vi "TDMS_Open - 1D.vi"(7 "Offset":bool, 8 "Gate 2":dbl=15.0, 9 "Gate 1":dbl=5.0, 10 "Input 2D":dbl[][](array[numeric]), 11 "Open":bool) -> (1 "Output 2D":dbl[][](array[numeric]), 3 "Freq_Sampling_SizeX_SizeY":dbl[](array[numeric]))   [LabVIEW 2018]
uses:
  <vilib>/Platform/NI_3dgraph.lvlib
panel:
  in  "milliseconds to wait":u32
  in  "3D Surface":refnum<k7>(container)
  in  "Samples per Channel":i32=1000 caption="Samples"
  in  "Rate":dbl=60000.0 caption="Sample Rate (Hz)" format="%0.0f"
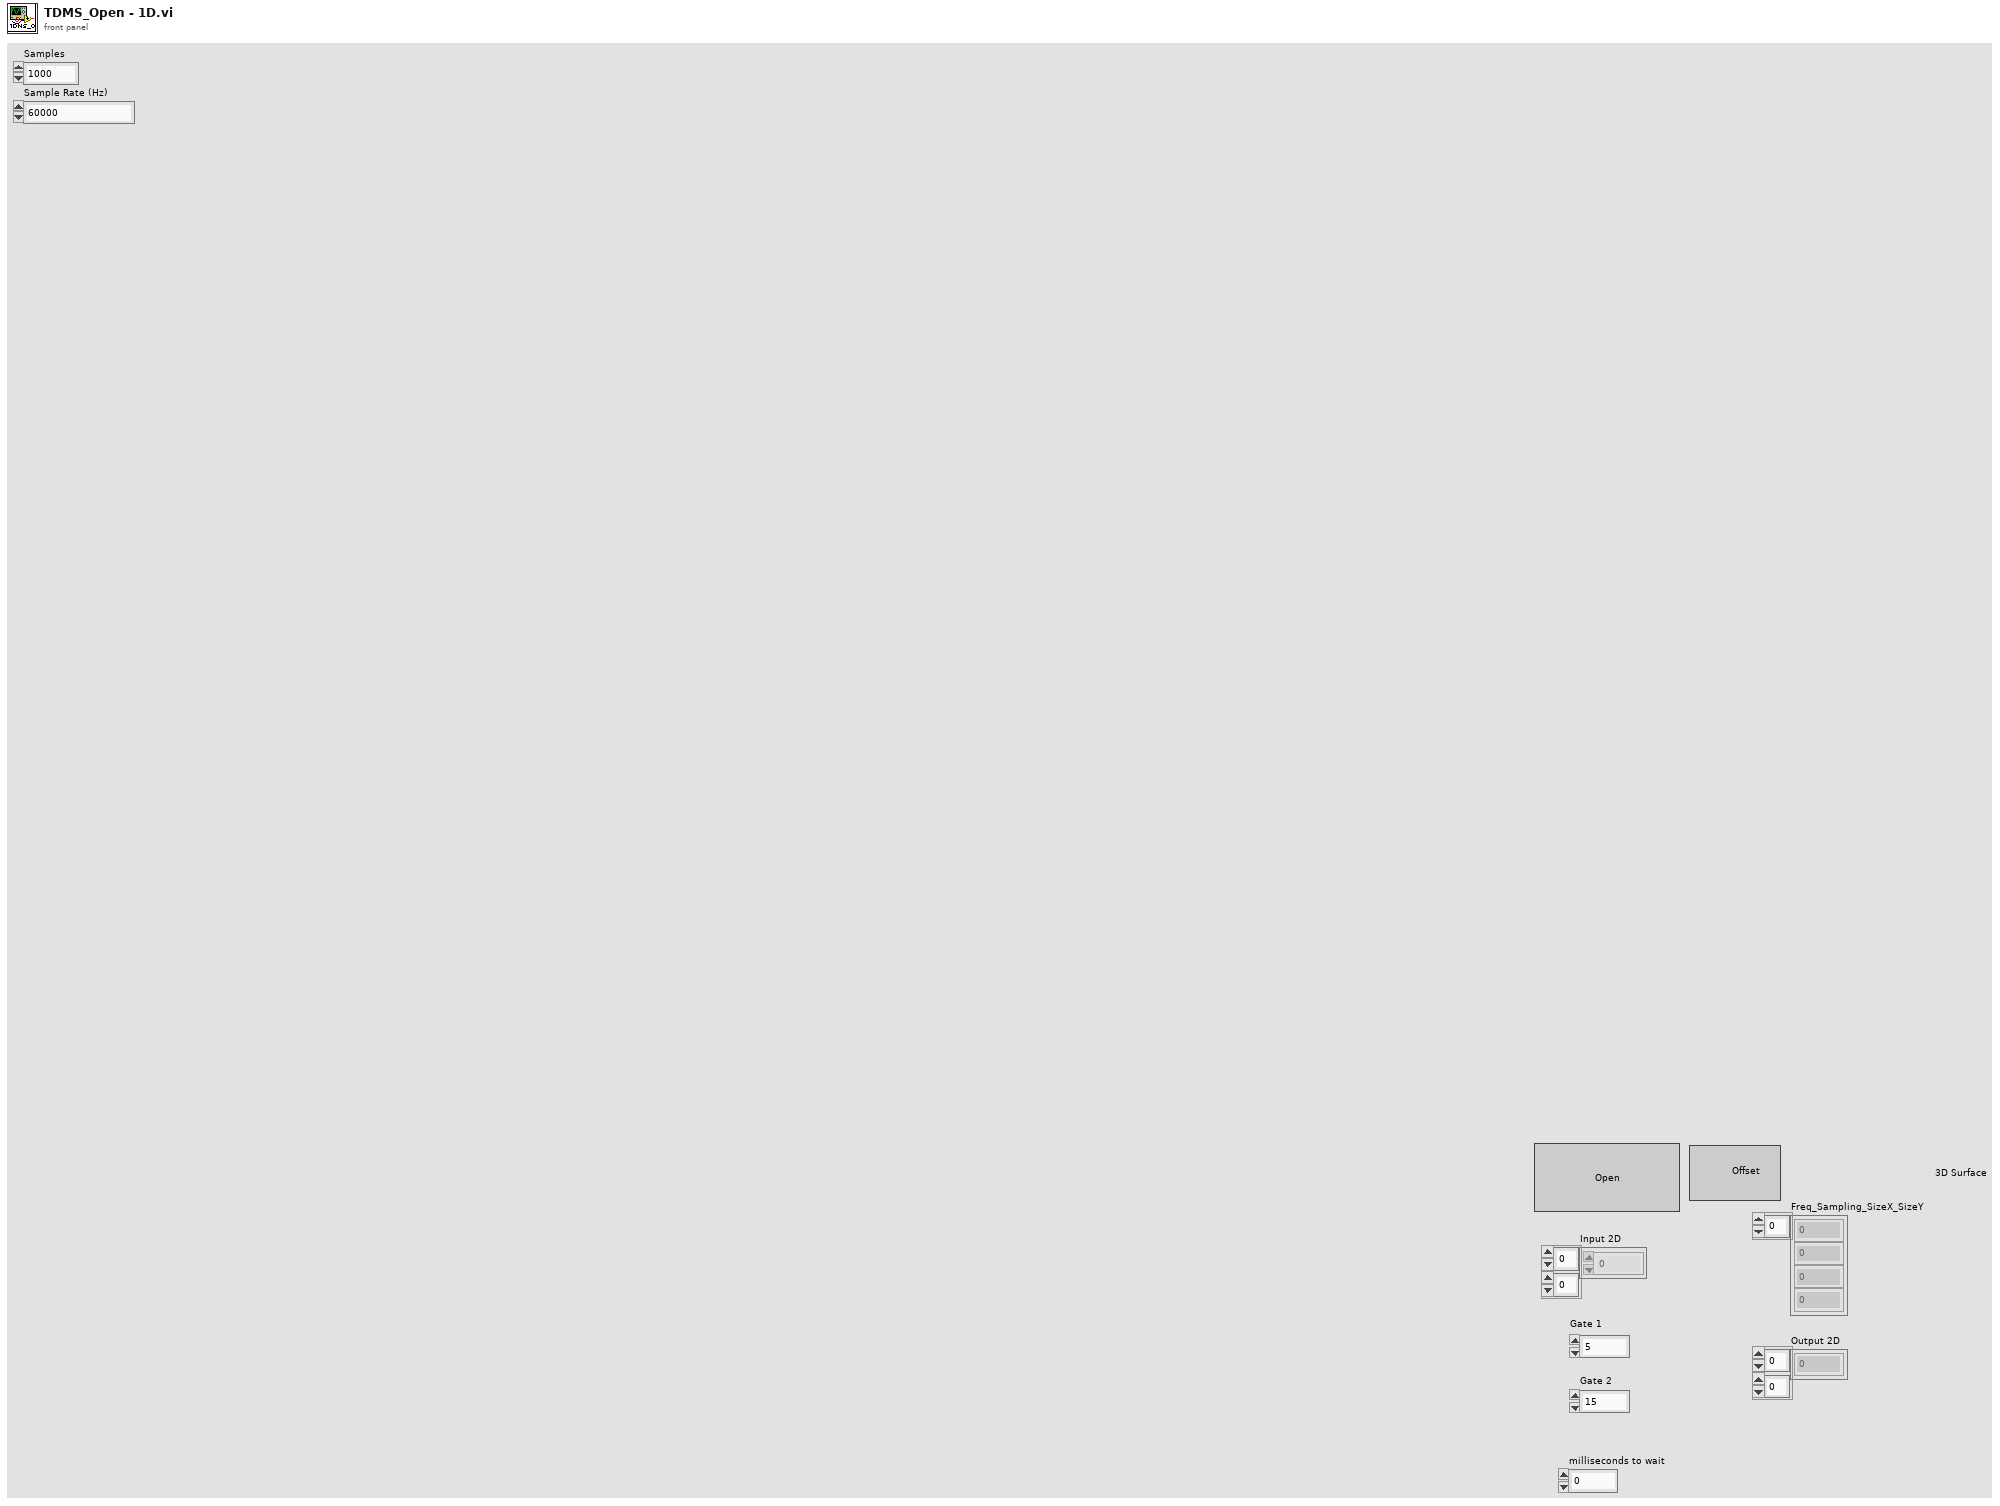
[diagram p1: front panel]
types:
  T1 = enum16{"open", "open or create", "create or replace", "create", "open (read-only)"}
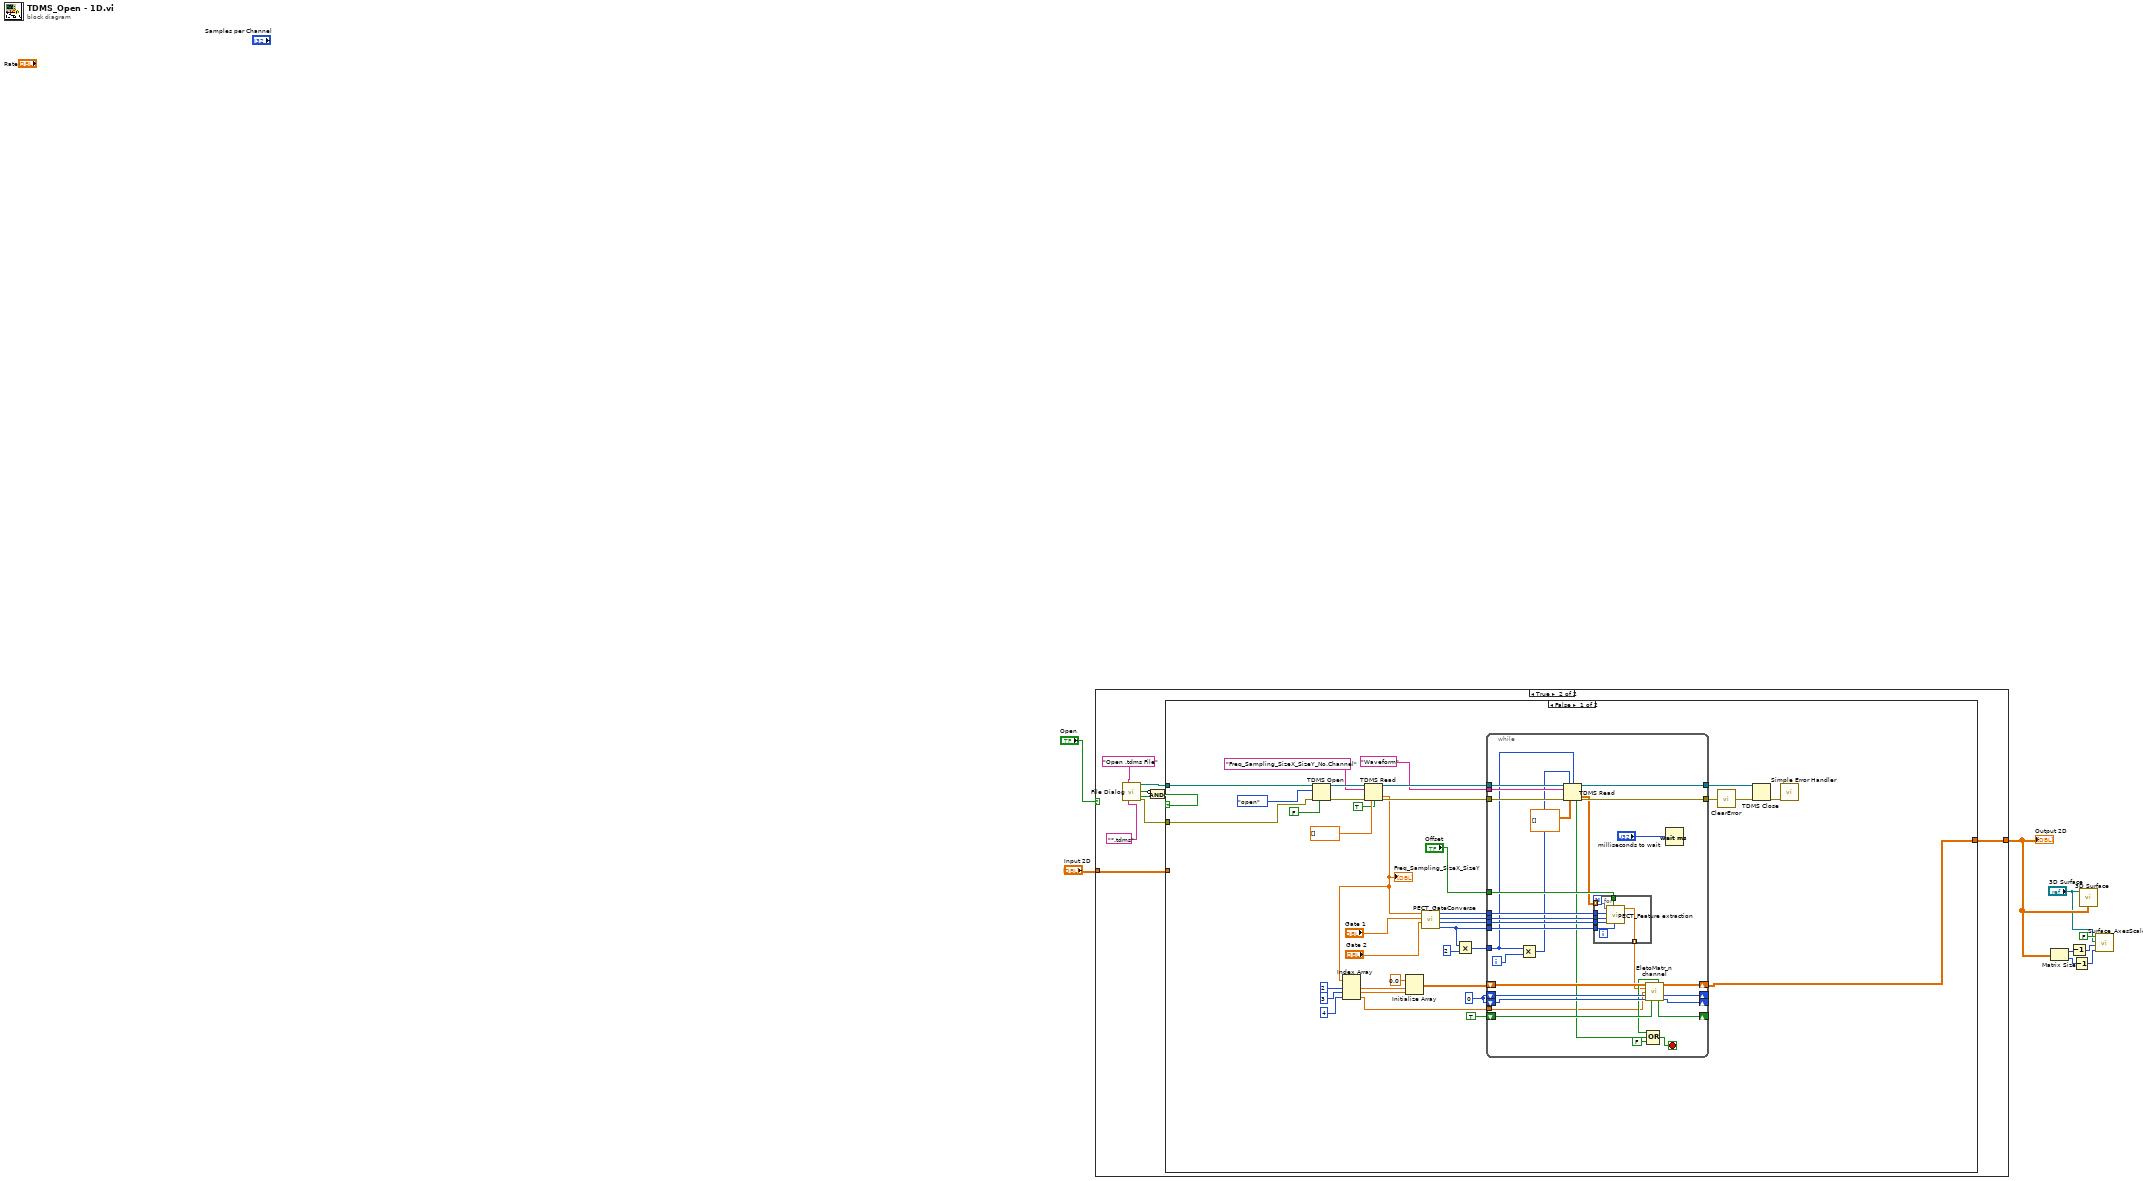
[diagram p0: block diagram]
diagram:
  n1 = case shown="True" "Open" {
    tunnel: [w10 w13] -> w4
    tunnel: "Input 2D" -> [w10 w12]
    frame False {
    }
    frame True {
      n2 = call "File Dialog"("prompt"="Open .tdms File" ("button label"), "pattern (all files)"="*.tdms") -> ("selected path"=w19:path, "exists"=w17:bool, "cancelled"=w16:bool, "error out"=w11:errorcluster)  [unwired: 10 in]
      n3 = Compound Arithmetic op=AND(invert w17, w16) -> (w15:bool)
      n4 = case shown="False" w15 {
        tunnel: w19 -> [w24 _]
        tunnel: [w22 w94] -> w13
        tunnel: w12 -> [_ w94]
        tunnel: w11 -> [w46 _]
        frame False {
          w33 = 0 ("Out Row")
          n5 = TDMS Open(6:FALSE ("disable buffering (T)"), 8:w46, 10:T1."open" ("operation"), 11:w24) -> (0:w52:errorcluster, 3:w56:refnum<k34>)  [unwired: 3 in]
          n6 = TDMS Read(0:w56, 5:"Freq_Sampling_SizeX_SizeY_No.Channel" ("group name in"), 11:w52, 12:dbl[] [] ("Array"), 13:TRUE ("return channels in file order? (F)")) -> (4:w28:refnum<k34>, 10:w23:dbl[], 15:w45:errorcluster)  [unwired: 3 in, 3 out]
          "Freq_Sampling_SizeX_SizeY" <- w23
          n7 = Index Array(array=w23, index #1=2 ("index"), index #2=3 ("index"), index #3=4 ("index")) -> (element #1=w35:dbl, element #2=w34:dbl, element #3=w20:dbl)
          n8 = Initialize Array(0.0 ("element"), w35, w34) -> (w36:dbl[][])
          n9 = call "PECT_GateConverse.vi"("Gate 2"="Gate 2", "Gate 1"="Gate 1", "Freq_Sampling_SizeX_SizeY"=w23) -> ("Length T/2"=w30:i32, "Length"=w40:i32, "Start 2"=w41:i32, "Start 1"=w42:i32)  [unwired: 4 in, 1 out]
          n10 = Multiply(x=w30, y=2) -> (x*y=w29:i32)
          n11 = while {
            tunnel: [w86] -> w48
            tunnel: [w85] -> w47
            tunnel: "Waveform" ("group name in") -> [w66]
            tunnel: w28 -> [w83]
            tunnel: w45 -> [w82]
            tunnel: w42 -> [w81]
            tunnel: w41 -> [w80]
            tunnel: w40 -> [w79]
            shift-right: [w77] -> w22
            shift-left: w36 -> [w78]
            shift-right: [w74] -> _
            shift-left: w33 -> [w76]
            shift-right: [w73] -> _
            shift-left: w33 -> [w75]
            shift-right: [w71] -> _
            shift-left: TRUE ("Output Direction") -> [w72]
            tunnel: w29 -> [w64]
            tunnel: w30 -> [w70]
            tunnel: "Offset" -> [w67]
            tunnel: w20 -> [w57]
            i -> [w68]
            stop <- w60 stop-if-true
            n12 = Multiply(x=w64, y=w68) -> (x*y=w65:i32)
            n13 = TDMS Read(0:w83, 1:w65, 2:w64, 5:w66, 11:w82, 12:dbl[][] [] ("Array")) -> (4:w86:refnum<k34>, 10:w63:dbl[][], 14:w61:bool, 15:w85:errorcluster)  [unwired: 2 in, 2 out]
            n14 = for {
              tunnel: w81 -> [w93]
              tunnel: w80 -> [w92]
              tunnel: w79 -> [w91]
              tunnel: [w90] -> w58 mode=indexing
              tunnel: w70 -> [w89]
              tunnel: w67 -> [w88]
              tunnel: w63 -> [w87] mode=indexing
              n15 = call "PECT_Feature extraction.vi"("Length T/2"=w89, "Offset"=w88, "Length"=w91, "Start 2"=w92, "Start 1"=w93, "Pulse signal in"=w87) -> ("Feature extraction out"=w90:dbl)  [unwired: 5 in]
            }
            n16 = call "EletoMatr_n channel.vi"("Input Array X"=w78, "Input data"=w58, "No. channels"=w57, "In Row"=w76, "In Column"=w75, "Input Direction"=w72) -> ("Completed"=w62:bool, "Out Array X"=w77:dbl[][], "Out Row"=w74:i32, "Output Direction"=w71:bool, "Out Column"=w73:i32)  [unwired: 5 in]
            n17 = Compound Arithmetic op=OR(w62, w61, FALSE ("value")) -> (w60:bool)
            n18 = Wait (ms)(milliseconds to wait="milliseconds to wait") -> ()  [unwired: 1 out]
          }
          n19 = call <vilib>:"ClearError.vi"("error in (no error)"=w47) -> ("error out"=w50:errorcluster)
          n20 = TDMS Close(8:w50, 11:w48) -> (0:w49:errorcluster)  [unwired: 1 out]
          n21 = call <vilib>:"Simple Error Handler.vi"("error in (no error)"=w49) -> ()  [unwired: 1 in, 8 out]
        }
        frame True {
        }
      }
    }
  }
  "Output 2D" <- w4
  n22 = Matrix Size(0:w4) -> (1:w5:i32, 2:w2:i32)
  n23 = Decrement(x=w5) -> (x-1=w7:i32)
  n24 = Decrement(x=w2) -> (x-1=w1:i32)
  n25 = call <vilib>:"3D Surface.vi"("z matrix"=w4, "3D graph"="3D Surface") -> ()  [unwired: 8 in, 2 out]
  n26 = call "Surface_AxesScale.vi"("Y-axis Max"=w1, "X-axis max"=w7, "3D Surface"="3D Surface", "Auto Scale"=FALSE) -> ()  [unwired: 8 in]
